vi "ex05_ITEM.vi"() -> ()   [LabVIEW 2011]
panel:
  in  "stop":bool
  out "Boolean":bool
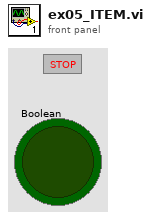
[diagram p1: front panel]
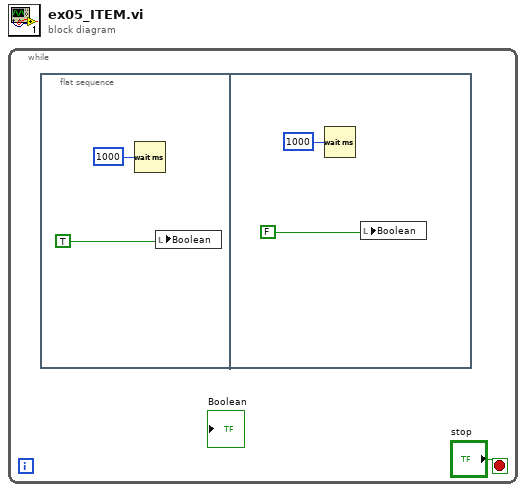
[diagram p0: block diagram]
diagram:
  n1 = while {
    stop <- "stop" stop-if-true
    n2 = flat-sequence {
      frame #0 {
        n3 = Wait (ms)(milliseconds to wait=u32 1000) -> ()  [unwired: 1 out]
        n4 = local write "Boolean"(TRUE) -> ()
      }
      frame #1 {
        n5 = Wait (ms)(milliseconds to wait=u32 1000) -> ()  [unwired: 1 out]
        n6 = local write "Boolean"(FALSE) -> ()
      }
    }
  }
